vi "ScanRevised_carter.vi"() -> ()   [LabVIEW 2023, in "HP4192A IA.lvclass"]
uses:
  HP4192A IA.lvclass
  <vilib>/Analysis/baseanly.llb/Mean (DBL).vi
  Global/GPIB Numbers.vi
  Global/Relative Sound Files.vi
  HP4192A Impedance Analyzer/HP4192 Impedance Analyzer.lvlib
  <vilib>/Analysis/NI_AALBase.lvlib
panel:
  in  "Tab Control":enum32{"Z", "R", "L", "C"}(tab)
  out "Impedance":cluster{"Y":dbl[], "Y":dbl[]}[](graph)=[{"Y"=[5.0, 5.0, 5.0, 5.0, 5.0], "Y"=[-246999.99999999997, -1063000.0, -361000.0, -401000.0, -539000.0]}]
  out "Resistance":cluster{"Y":dbl[], "Y":dbl[]}[](graph)=[{"Y"=[5.0, 5.0, 5.0, 5.0, 5.0], "Y"=[-246999.99999999997, -1063000.0, -361000.0, -401000.0, -539000.0]}]
  out "Inductance":cluster{"Y":dbl[], "Y":dbl[]}[](graph)=[{"Y"=[5.0, 5.0, 5.0, 5.0, 5.0], "Y"=[-246999.99999999997, -1063000.0, -361000.0, -401000.0, -539000.0]}]
  out "Capacitance":cluster{"Y":dbl[], "Y":dbl[]}[](graph)=[{"Y"=[5.0, 5.0, 5.0, 5.0, 5.0], "Y"=[-246999.99999999997, -1063000.0, -361000.0, -401000.0, -539000.0]}]
  out "Boolean 4":bool
  out "Boolean 3":bool
  out "Boolean 2":bool
  out "Boolean":bool
  in  "Numeric":i32=5
  out "dataTxt":string
  in  "Export\nPlot":bool
  in  "path":path
  out "error out":errorcluster
  in  "error in":errorcluster
  in  "Notes":string
  out "current numpoints":dbl
  in  "Take additional samples?":bool
  in  "number of samples in this range":i32=101
  in  "end freq for add'l sample":dbl[unit]=13000000.0
  in  "start freq for add'l samples":dbl[unit]=5.0
  in  "Total number of freq points":dbl=101.0
  in  "Final frequency":dbl[unit]=13000000.0
  in  "Initial frequency":dbl[unit]=5.0
  in  "Averaging?":bool
  in  "Delay between\nsteps (ms)":u32=500
  in  "stop":bool
  out "Current Frequency":dbl[unit]
  in  "start":bool
  in  "L":bool
  in  "C":bool
  in  "R":bool
  in  "Z":bool
  # "Measure"
  # "Frequency range for additional samples"
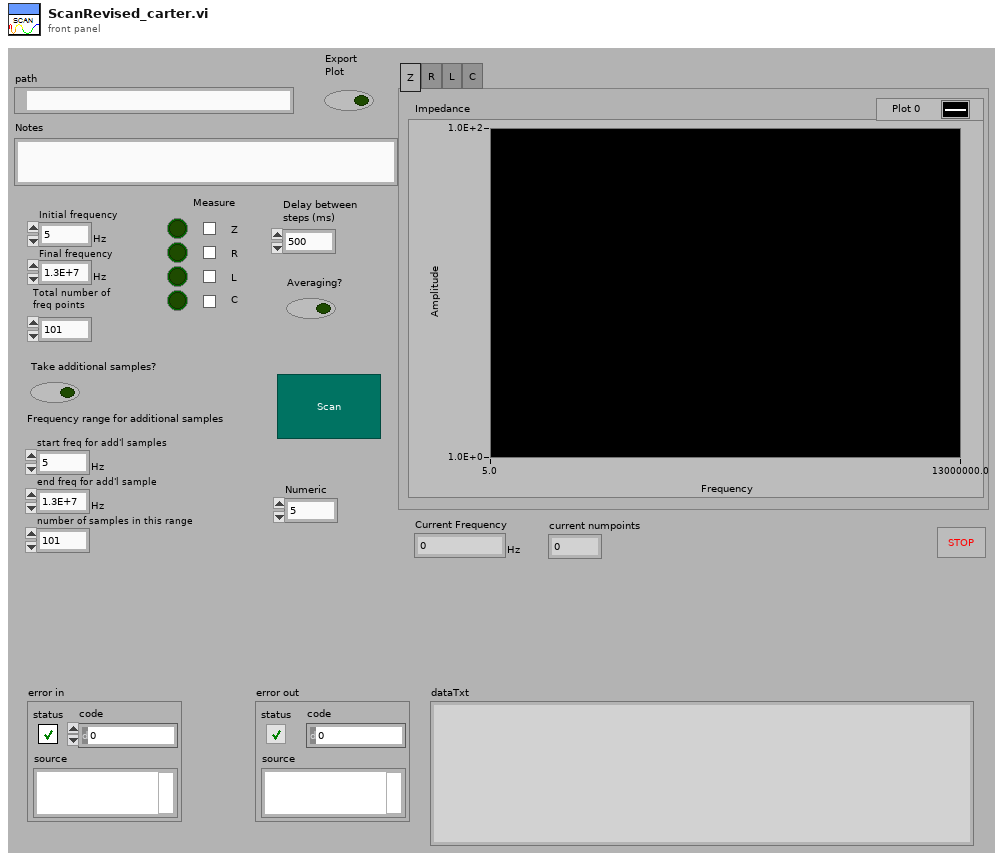
[diagram p1: front panel]
types:
  T1 = typedef "GPIB Type Def.ctl" = cluster{"Name":string, "bus":dbl, "GPIB":dbl, "GPIB as string":string, "byte":i32, "VISA Resource Name":refnum<visa-resource-name>}
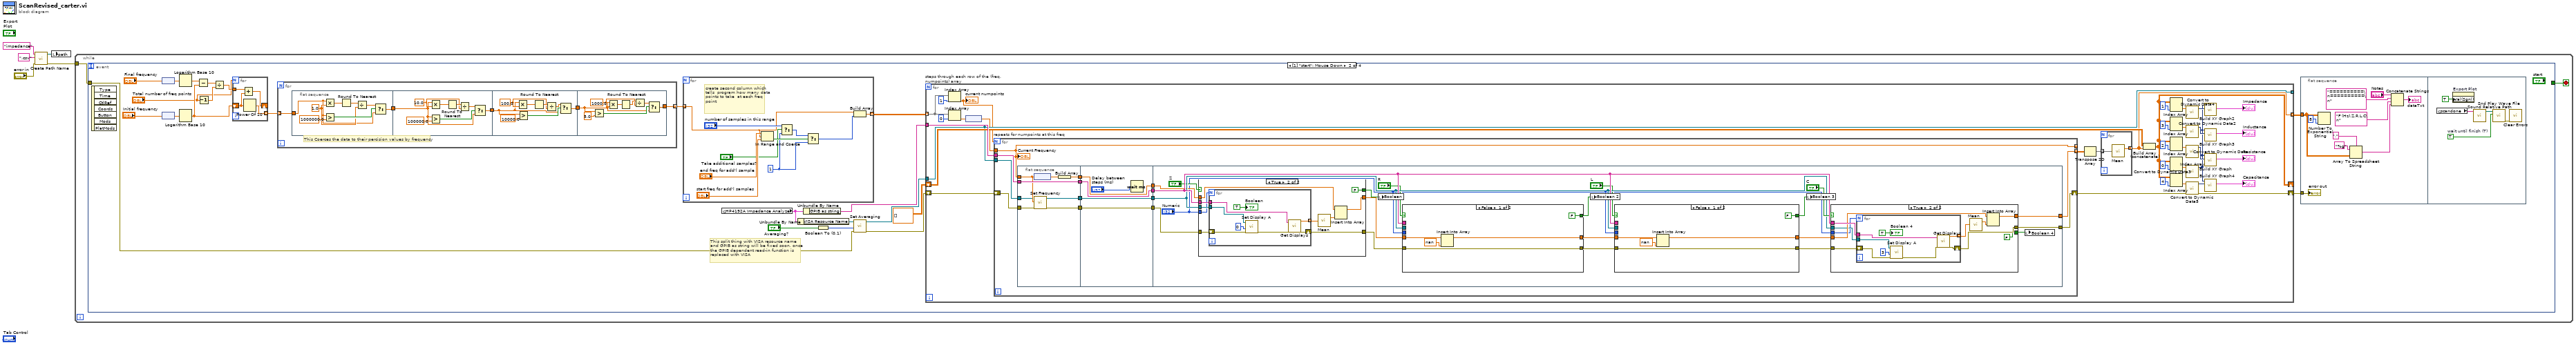
[diagram p0: block diagram]
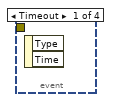
[diagram p2: hidden frame]
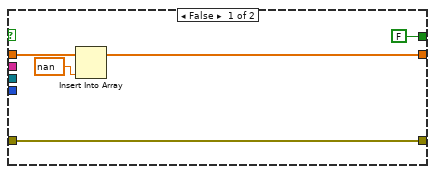
[diagram p3: hidden frame]
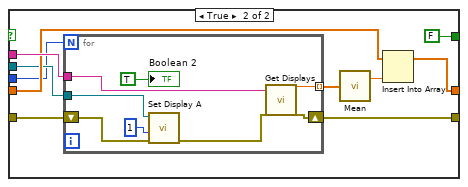
[diagram p4: hidden frame]
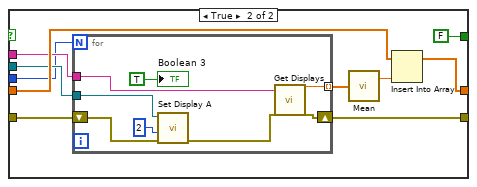
[diagram p5: hidden frame]
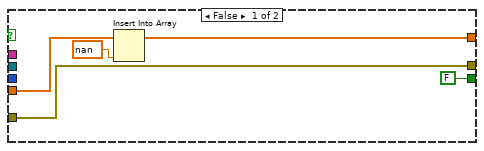
[diagram p6: hidden frame]
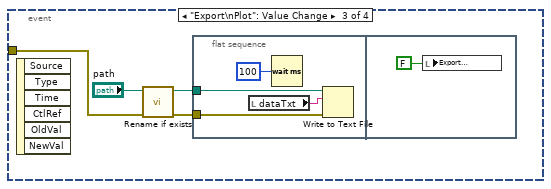
[diagram p7: hidden frame]
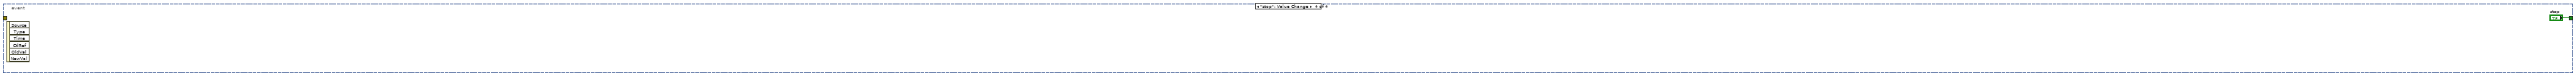
[diagram p8: hidden frame]
diagram:
  n1 = call "Create Path Name.vi"("error in"="error in", "String"=".csv", "filename"="impedance") -> ("error out"=w2:errorcluster, "path"=w4:path)  [unwired: 3 out]
  n2 = local write "path"(w4) -> ()
  n3 = while {
    tunnel: w2 -> [w6]
    stop <- w7 stop-if-true
    n4 = event shown="[1] \"start\": Mouse Down" {
      selector: _ -> [_ _ _ _]
      dyn-events: _ -> [_ _ _ _]
      timeout: _ -> [_ _ _ _]
      tunnel: [_ _ _ "stop"] -> w7
      tunnel: w6 -> [_ w11 w276 _]
      event Timeout {
        n5 = event-data() -> ()  [unwired: 1 in, 2 out]
      }
      event "start": Mouse Down {
        # "This split thing with VISA resource name  \nand GPIB as string will be fixed soon, once\nthe GPIB dependent read-in function is\nreplaced with VISA"
        n6 = event-data() -> ()  [unwired: 1 in, 7 out]
        n7 = node("Final frequency") -> (w19:dbl)
        n8 = node("Initial frequency") -> (w21:dbl)
        n9 = Logarithm Base 10(1:w19) -> (0:w26:dbl)
        n10 = Logarithm Base 10(1:w21) -> (0:w25:dbl)
        n11 = Subtract(x=w26, y=w25) -> (x-y=w31:dbl)
        n12 = Decrement(x="Total number of freq points") -> (x-1=w24:dbl)
        n13 = Divide(x=w31, y=w24) -> (x/y=w30:dbl)
        n14 = for {
          N: "Total number of freq points" -> [_]
          shift-right: [w273] -> _
          shift-left: w25 -> [w271]
          tunnel: w30 -> [w272]
          tunnel: [w270] -> w9 mode=indexing
          n15 = Add(x=w272, y=w271) -> (x+y=w273:dbl)
          n16 = Power Of 10(x=w271) -> (10^x=w270:dbl)
        }
        n17 = for {
          tunnel: w9 -> [w36] mode=indexing
          tunnel: [w35] -> w8 mode=indexing
          # "This Coerces the data to their percision values by frequency"
          n18 = flat-sequence {
            tunnel: w36 -> [w38]
            tunnel: [w37] -> w34
            tunnel: w34 -> [w46]
            tunnel: [w45] -> w33
            tunnel: w33 -> [w54]
            tunnel: [w53] -> w32
            tunnel: [w61] -> w35
            tunnel: w32 -> [w62]
            frame #0 {
              w41 = 1.0 ("y")
              n19 = Multiply(x=w38, y=w41) -> (x*y=w42:dbl)
              n20 = Greater?(x=w38, y=1000000.0) -> (0:w43:bool)
              n21 = Round To Nearest(number=w42) -> (nearest integer value=w40:dbl)
              n22 = Divide(x=w40, y=w41) -> (x/y=w39:dbl)
              n23 = Select(t=w39, s=w43, f=w38) -> (s? t:f=w37:dbl)
            }
            frame #1 {
              w47 = 10.0 ("y")
              n24 = Multiply(x=w46, y=w47) -> (x*y=w50:dbl)
              n25 = Greater?(x=w46, y=100000.0) -> (0:w49:bool)
              n26 = Round To Nearest(number=w50) -> (nearest integer value=w51:dbl)
              n27 = Divide(x=w51, y=w47) -> (x/y=w52:dbl)
              n28 = Select(t=w52, s=w49, f=w46) -> (s? t:f=w45:dbl)
            }
            frame #2 {
              w55 = 100.0 ("y")
              n29 = Multiply(x=w54, y=w55) -> (x*y=w58:dbl)
              n30 = Greater?(x=w54, y=10000.0) -> (0:w57:bool)
              n31 = Round To Nearest(number=w58) -> (nearest integer value=w59:dbl)
              n32 = Divide(x=w59, y=w55) -> (x/y=w60:dbl)
              n33 = Select(t=w60, s=w57, f=w54) -> (s? t:f=w53:dbl)
            }
            frame #3 {
              w63 = 1000.0 ("y")
              n34 = Greater?(x=w62, y=5.0) -> (0:w65:bool)
              n35 = Multiply(x=w62, y=w63) -> (x*y=w66:dbl)
              n36 = Round To Nearest(number=w66) -> (nearest integer value=w67:dbl)
              n37 = Divide(x=w67, y=w63) -> (x/y=w68:dbl)
              n38 = Select(t=w68, s=w65, f=w62) -> (s? t:f=w61:dbl)
            }
          }
        }
        n39 = for {
          tunnel: w8 -> [w260] mode=indexing
          tunnel: [w261] -> w18 mode=indexing
          w264 = 1 ("f")
          # "create second column which tells  program how many data points to take  at each freq point"
          n40 = In Range and Coerce(upper limit="end freq for add'l sample", x=w260, lower limit="start freq for add'l samples") -> (In Range?=w267:bool)  [unwired: 1 out]
          n41 = Select(t="number of samples in this range", s="Take additional samples?", f=w264) -> (s? t:f=w263:i32)
          n42 = Select(t=w263, s=w267, f=w264) -> (s? t:f=w262:i32)
          n43 = Build Array(w260, w262) -> (w261:dbl[])
        }
        n44 = global read "GPIB Numbers.vi" "HP4192A Impedance Analyzer"() -> (w27:T1)
        n45 = Unbundle By Name(w27) -> ("VISA Resource Name"=w28:refnum<visa-resource-name>)
        n46 = Unbundle By Name(w27) -> ("GPIB as string"=w29:string)
        n47 = Boolean To (0,1)(Boolean="Averaging?") -> (0, 1=w15:i16)
        n48 = call "Set Averaging.vi"("error in (no error)"=w11, "Averaging"=w15, "VISA resource name"=w28) -> ("error out"=w13:errorcluster, "VISA resource name out"=w14:refnum<visa-resource-name>)  [unwired: 7 in]
        n49 = for "steps through each row of the (freq, numpoints) array" {
          tunnel: w18 -> [w106] mode=indexing
          tunnel: w29 -> [w117]
          tunnel: [w100] -> w10 mode=indexing
          shift-right: [w87] -> _
          shift-left: dbl[][] [] -> [w116]
          tunnel: [w115] -> _ mode=indexing
          tunnel: w14 -> [w115]
          shift-right: [w98] -> w12
          shift-left: w13 -> [w99]
          n50 = Index Array(array=w106, index=1) -> (element=w108:dbl)
          "current numpoints" <- w108
          n51 = Index Array(array=w106, index=0) -> (element=w104:dbl)
          n52 = node(w104) -> (w103:dbl[unit])
          n53 = for "repeats for numpoints at this freq" {
            N: w108 -> [_]
            tunnel: w117 -> [w127]
            tunnel: w103 -> [w120]
            tunnel: [w126] -> w102 mode=indexing
            tunnel: w115 -> [w125]
            shift-right: [w121] -> w98
            shift-left: w99 -> [w124]
            tunnel: [w120] -> _ mode=indexing
            n54 = flat-sequence {
              tunnel: w127 -> [w139]
              tunnel: [w139] -> w133
              tunnel: w120 -> [w138]
              tunnel: [w141] -> w132
              tunnel: w125 -> [w137]
              tunnel: [w136] -> w131
              tunnel: w124 -> [w135]
              tunnel: [w134] -> w122
              tunnel: w133 -> [w145]
              tunnel: [w145] -> w130
              tunnel: w132 -> [w144]
              tunnel: [w144] -> w129
              tunnel: [w143] -> w128
              tunnel: w131 -> [w143]
              tunnel: [w142] -> w123
              tunnel: w122 -> [w142]
              tunnel: [w165] -> w126
              tunnel: [w161] -> w121
              tunnel: w123 -> [w153]
              tunnel: w128 -> [w163]
              tunnel: w129 -> [w155]
              tunnel: w130 -> [w167]
              frame #0 {
                n55 = node(w138) -> (w140:dbl)
                n56 = call "Set Frequency.vi"("error in (no error)"=w135, "test signal freq"=w138, "VISA resource name"=w137) -> ("error out"=w134:errorcluster, "VISA resource name out"=w136:refnum<visa-resource-name>)  [unwired: 7 in]
                n57 = Build Array(w140) -> (w141:dbl[])
              }
              frame #1 {
                n58 = Wait (ms)(milliseconds to wait="Delay between\nsteps (ms)") -> ()  [unwired: 1 out]
              }
              frame #2 {
                n59 = case shown="True" "Z" {
                  tunnel: w155 -> [w170 w181]
                  tunnel: w167 -> [_ w182]
                  tunnel: [w169 w180] -> w157
                  tunnel: w163 -> [_ w176]
                  tunnel: w153 -> [w172 w177]
                  tunnel: [w172 w175] -> w152
                  tunnel: "Numeric" -> [_ w174]
                  tunnel: [FALSE ("Boolean") FALSE ("Boolean")] -> w150
                  frame False {
                    n60 = Insert Into Array(array=w170, new element=nan) -> (w169:dbl[])  [unwired: 1 in]
                  }
                  frame True {
                    n61 = for {
                      N: w174 -> [_]
                      tunnel: w182 -> [w190]
                      tunnel: [w189] -> w179 mode=indexing
                      tunnel: w176 -> [w187]
                      shift-right: [w185] -> w175
                      shift-left: w177 -> [w188]
                      n62 = call "Set Display A.vi"("error in (no error)"=w188, "function A (z/y:0)"=i16 0, "VISA resource name"=w187) -> ("error out 2"=w186:errorcluster)  [unwired: 8 in]
                      n63 = call "Get Displays.vi"("GPIB addess"=w190, "error in (no error)"=w186) -> ("display A"=w189:dbl, "error out"=w185:errorcluster)  [unwired: 17 in, 7 out]
                      "Boolean" <- TRUE ("Boolean")
                    }
                    n64 = call-poly <vilib>:"Mean.vi"("X"=w179) -> ("mean"=w178:dbl)  [unwired: 1 out]
                    n65 = Insert Into Array(array=w181, new element=w178) -> (w180:dbl[])  [unwired: 1 in]
                  }
                }
                n66 = local write "Boolean"(w150) -> ()
                n67 = case shown="False" "R" {
                  tunnel: w167 -> [_ w205]
                  tunnel: w157 -> [w191 w204]
                  tunnel: [w192 w203] -> w160
                  tunnel: w163 -> [_ w202]
                  tunnel: w152 -> [w195 w201]
                  tunnel: [w195 w200] -> w158
                  tunnel: "Numeric" -> [_ w197]
                  tunnel: [FALSE ("Boolean 2") FALSE ("Boolean 2")] -> w149
                  frame False {
                    n68 = Insert Into Array(array=w191, new element=nan ("new element/subarray")) -> (w192:dbl[])  [unwired: 1 in]
                  }
                  frame True {
                    n69 = for {
                      N: w197 -> [_]
                      tunnel: [w213] -> w199 mode=indexing
                      tunnel: w205 -> [w212]
                      tunnel: w202 -> [w211]
                      shift-right: [w208] -> w200
                      shift-left: w201 -> [w210]
                      n70 = call "Set Display A.vi"("error in (no error)"=w210, "function A (z/y:0)"=i16 1, "VISA resource name"=w211) -> ("error out 2"=w209:errorcluster)  [unwired: 8 in]
                      n71 = call "Get Displays.vi"("GPIB addess"=w212, "error in (no error)"=w209) -> ("display A"=w213:dbl, "error out"=w208:errorcluster)  [unwired: 17 in, 7 out]
                      "Boolean 2" <- TRUE ("Boolean 2")
                    }
                    n72 = call-poly <vilib>:"Mean.vi"("X"=w199) -> ("mean"=w198:dbl)  [unwired: 1 out]
                    n73 = Insert Into Array(array=w204, new element=w198) -> (w203:dbl[])  [unwired: 1 in]
                  }
                }
                n74 = local write "Boolean 2"(w149) -> ()
                n75 = case shown="False" "L" {
                  tunnel: [w215 w228] -> w166
                  tunnel: w160 -> [w216 w227]
                  tunnel: w167 -> [_ w226]
                  tunnel: w163 -> [_ w225]
                  tunnel: w158 -> [w218 w224]
                  tunnel: [w218 w223] -> w162
                  tunnel: "Numeric" -> [_ w220]
                  tunnel: [FALSE ("Boolean 3") FALSE ("Boolean 3")] -> w148
                  frame False {
                    n76 = Insert Into Array(array=w216, new element=nan) -> (w215:dbl[])  [unwired: 1 in]
                  }
                  frame True {
                    n77 = for {
                      N: w220 -> [_]
                      tunnel: [w236] -> w222 mode=indexing
                      tunnel: w226 -> [w235]
                      tunnel: w225 -> [w234]
                      shift-right: [w231] -> w223
                      shift-left: w224 -> [w233]
                      n78 = call "Set Display A.vi"("error in (no error)"=w233, "function A (z/y:0)"=i16 2, "VISA resource name"=w234) -> ("error out 2"=w232:errorcluster)  [unwired: 8 in]
                      n79 = call "Get Displays.vi"("GPIB addess"=w235, "error in (no error)"=w232) -> ("display A"=w236:dbl, "error out"=w231:errorcluster)  [unwired: 17 in, 7 out]
                      "Boolean 3" <- TRUE ("Boolean 3")
                    }
                    n80 = call-poly <vilib>:"Mean.vi"("X"=w222) -> ("mean"=w221:dbl)  [unwired: 1 out]
                    n81 = Insert Into Array(array=w227, new element=w221) -> (w228:dbl[])  [unwired: 1 in]
                  }
                }
                n82 = local write "Boolean 3"(w148) -> ()
                n83 = case shown="True" "C" {
                  tunnel: [w238 w251] -> w165
                  tunnel: w167 -> [_ w250]
                  tunnel: w166 -> [w239 w249]
                  tunnel: w163 -> [_ w248]
                  tunnel: w162 -> [w241 w247]
                  tunnel: [w241 w246] -> w161
                  tunnel: "Numeric" -> [_ w243]
                  tunnel: [FALSE ("Boolean 3") FALSE ("Boolean 3")] -> w147
                  frame False {
                    n84 = Insert Into Array(array=w239, new element=nan) -> (w238:dbl[])  [unwired: 1 in]
                  }
                  frame True {
                    n85 = for {
                      N: w243 -> [_]
                      tunnel: [w259] -> w245 mode=indexing
                      tunnel: w250 -> [w258]
                      tunnel: w248 -> [w257]
                      shift-right: [w254] -> w246
                      shift-left: w247 -> [w256]
                      n86 = call "Set Display A.vi"("error in (no error)"=w256, "function A (z/y:0)"=i16 3, "VISA resource name"=w257) -> ("error out 2"=w255:errorcluster)  [unwired: 8 in]
                      n87 = call "Get Displays.vi"("GPIB addess"=w258, "error in (no error)"=w255) -> ("display A"=w259:dbl, "error out"=w254:errorcluster)  [unwired: 17 in, 7 out]
                      "Boolean 4" <- TRUE ("Boolean 3")
                    }
                    n88 = call-poly <vilib>:"Mean.vi"("X"=w245) -> ("mean"=w244:dbl)  [unwired: 1 out]
                    n89 = Insert Into Array(array=w249, new element=w244) -> (w251:dbl[])  [unwired: 1 in]
                  }
                }
                n90 = local write "Boolean 4"(w147) -> ()
              }
            }
            "Current Frequency" <- w120
          }
          n91 = Transpose 2D Array(2D array=w102) -> (transposed array=w101:dbl[][])
          n92 = for {
            tunnel: w101 -> [w119] mode=indexing
            tunnel: [w118] -> w100 mode=indexing
            n93 = call-poly <vilib>:"Mean.vi"("X"=w119) -> ("mean"=w118:dbl)  [unwired: 1 out]
          }
          n94 = Build Array (concatenate)(w116, w100) -> (w87:dbl[][])
          n95 = Index Array(array=w87, index (col)=1) -> (element=w109:dbl[])  [unwired: 1 in]
          n96 = Index Array(array=w87, index (col)=3) -> (element=w91:dbl[])  [unwired: 1 in]
          n97 = Index Array(array=w87, index (col)=2) -> (element=w95:dbl[])  [unwired: 1 in]
          n98 = Index Array(array=w87, index (col)=0) -> (element=w110:dbl[])  [unwired: 1 in]
          n99 = Index Array(array=w87, index (col)=4) -> (element=w88:dbl[])  [unwired: 1 in]
          n100 = call "Convert to Dynamic Data4"("Array"=w109) -> ("Dynamic Data Type"=w111:dynamicdata)  [unwired: 3 in]
          n101 = call "Convert to Dynamic Data2"("Array"=w91) -> ("Dynamic Data Type"=w92:dynamicdata)  [unwired: 3 in]
          n102 = call "Convert to Dynamic Data"("Array"=w95) -> ("Dynamic Data Type"=w96:dynamicdata)  [unwired: 3 in]
          n103 = call "Convert to Dynamic Data3"("Array"=w110) -> ("Dynamic Data Type"=w86:dynamicdata)  [unwired: 3 in]
          n104 = call "Convert to Dynamic Data5"("Array"=w88) -> ("Dynamic Data Type"=w89:dynamicdata)  [unwired: 3 in]
          n105 = call "Build XY Graph2"("Y Input"=w111, "X Input"=w86) -> ("XY Graph"=→"Impedance":cluster{"Y":dbl[], "Y":dbl[]}[])  [unwired: 8 in, 1 out]
          n106 = call "Build XY Graph3"("Y Input"=w92, "X Input"=w86) -> ("XY Graph"=→"Inductance":cluster{"Y":dbl[], "Y":dbl[]}[])  [unwired: 8 in, 1 out]
          n107 = call "Build XY Graph"("Y Input"=w96, "X Input"=w86) -> ("XY Graph"=→"Resistance":cluster{"Y":dbl[], "Y":dbl[]}[])  [unwired: 8 in, 1 out]
          n108 = call "Build XY Graph4"("Y Input"=w89, "X Input"=w86) -> ("XY Graph"=→"Capacitance":cluster{"Y":dbl[], "Y":dbl[]}[])  [unwired: 8 in, 1 out]
        }
        n109 = flat-sequence {
          tunnel: w12 -> [w78]
          tunnel: w10 -> [w70]
          frame #0 {
            n110 = Number To Exponential String(number=w70, precision (6)=i16 8) -> ()  [unwired: 2 in, 1 out]
            n111 = Array To Spreadsheet String(delimiter (Tab)=",", array=w70, 3:"%g") -> (spreadsheet string=w72:string)
            n112 = Concatenate Strings("Notes", "==========\n==========\n" ("string"), "F (Hz),Z,R,L,C\n", w72) -> (→"dataTxt":string)
            "error out" <- w78
          }
          frame #1 {
            w80 = TRUE  # wait until finish (T)
            n113 = global read "Relative Sound Files.vi" "scandone"() -> (w83:string)
            n114 = property on="Export Plot" class="Bool (strict)"("Val(Sgnl)"=TRUE ("Value (Signaling)")) -> ()  [unwired: 2 in, 2 out]
            n115 = call "Sound Relative Path.vi"("Sound"=w83) -> ("Relative Path"=w82:path)  [unwired: 10 in]
            n116 = call <vilib>:"Snd Play Wave File.vi"("wait until finish (T)"=w80, "wave file path"=w82) -> ("error out"=w81:errorcluster)  [unwired: 1 in, 8 out]
            n117 = call <vilib>:"Clear Errors.vi"("error in (no error)"=w81) -> ()  [unwired: 1 in, 6 out]
          }
        }
      }
      event "Export\nPlot": Value Change {
        n118 = event-data() -> ()  [unwired: 1 in, 6 out]
        n119 = call "Rename if exists.vi"("error in"=w276, "File Path"="path") -> ("error out"=w274:errorcluster, "New path"=w275:path)  [unwired: 1 in, 7 out]
        n120 = flat-sequence {
          tunnel: w275 -> [w280]
          tunnel: w274 -> [w279]
          frame #0 {
            n121 = local read "dataTxt"() -> (w281:string)
            n122 = Wait (ms)(milliseconds to wait=u32 100) -> ()  [unwired: 1 out]
            n123 = Write to Text File(file (use dialog)=w280, text=w281, error in=w279) -> ()  [unwired: 1 in, 3 out]
          }
          frame #1 {
            n124 = local write "Export\nPlot"(FALSE ("Export\nPlot")) -> ()
          }
        }
      }
      event "stop": Value Change {
        n125 = event-data() -> ()  [unwired: 1 in, 6 out]
      }
    }
  }
